vi "XYPlatform.vi"() -> ()   [LabVIEW 2017]
uses:
  <vilib>/Utility/error.llb/DialogType.ctl
  <vilib>/DAQmx/read.llb/DAQmx Read (Counter DBL 1Chan 1Samp).vi
  <vilib>/DAQmx/read.llb/DAQmx Read (Digital Bool 1Line 1Point).vi
  <vilib>/DAQmx/write.llb/DAQmx Write (Analog DBL 1Chan 1Samp).vi
  <vilib>/DAQmx/create/channels.llb/DAQmx Create Channel (AO-Voltage-Basic).vi
  <vilib>/DAQmx/create/channels.llb/DAQmx Create Channel (DI-Digital Input).vi
  <vilib>/DAQmx/create/channels.llb/DAQmx Create Channel (CI-Count Edges).vi
  <vilib>/functionblocks/Counter/Elapsed Timer/Elapsed Timer.vi
  <vilib>/DAQmx/miscellaneous.llb/DAQmx Fill In Error Info.vi
  <vilib>/functionblocks/FB Core/FB Core.xnode
  <vilib>/functionblocks/NI_FunctionBlock Libraries.lvlib
panel:
  in  "Zero":bool
  out "Dial Left Motor Voltage":dbl
  out "Dial Right Motor Voltage":dbl
  out "Left":bool
  out "Right":bool
  out "Down":bool
  out "Up":bool
  out "AngleLeft":bool
  out "RightIsStill":bool
  in  "Right Offset":dbl
  in  "Left Offset":dbl
  in  "Radius / cm":dbl
  out "Right Motor Pulses":dbl
  out "Left Motor Pulses":dbl
  in  "X position / cm":dbl(slide) scale=0.0..22.0
  in  "Y position / cm":dbl(slide) scale=0.0..14.0
  in  "Position Control":bool
  out "Y Position / cm":dbl
  out "X Position / cm":dbl
  in  "Draw Circle":bool
  out "Current Position":cluster{"Y":dbl[], "Y":dbl[]}[](graph)
  in  "X Voltage":dbl(slide) scale=-10.0..10.0
  in  "Y Voltage":dbl(slide) scale=-10.0..10.0
  in  "Home Button":bool=TRUE
  in  "Height / cm":dbl
  in  "Width / cm":dbl
  in  "Draw Rectangle":bool
  in  "Direction":sgl(knob)
  in  "Voltage of Dial":dbl
  out "Right Frequency (pulse/s)":dbl
  out "Left Frequency (pulse/s)":dbl
  out "Up Limit Switch":bool
  out "Down Limit Switch":bool
  out "Right Limit Switch":bool
  out "Left Limit Switch":bool
  in  "Left Motor Counter":tag="Dev5/ctr1"
  in  "Right Motor Counter":tag="Dev5/ctr0"
  in  "Left Limit Switch":tag="Dev5/port0/line3"
  in  "Right Limit Switch":tag="Dev5/port0/line2"
  in  "Down Limit Switch":tag="Dev5/port0/line1"
  in  "Up Limit Switch":tag="Dev5/port0/line0"
  in  "Motor Stop":bool
  in  "Left Motor":tag="Dev5/ao1"
  in  "Right Motor":tag="Dev5/ao0"
  in  "Min Voltage":dbl=-10.0
  in  "Max Voltage":dbl=10.0
  out "AngleRight":bool
  out "AngleDown":bool
  out "AngleUp":bool
  out "LeftIsStill":bool
  in  "Program Stop":bool
  out "Rectangle Right Ref":dbl
  out "Rectangle Left Ref":dbl
  out "Net Left Pulse":dbl
  out "Net Right Pulse":dbl
  out "Left Motor":dbl
  out "Right Motor":dbl
  out "Left Motor Pulses":dbl
  out "last left pulse":dbl format="%0.2f"
  out "Right Motor Pulses":dbl
  out "last right pulse":dbl format="%0.2f"
  out "Right Motor Timer":i32
  out "Left Motor Timer":i32
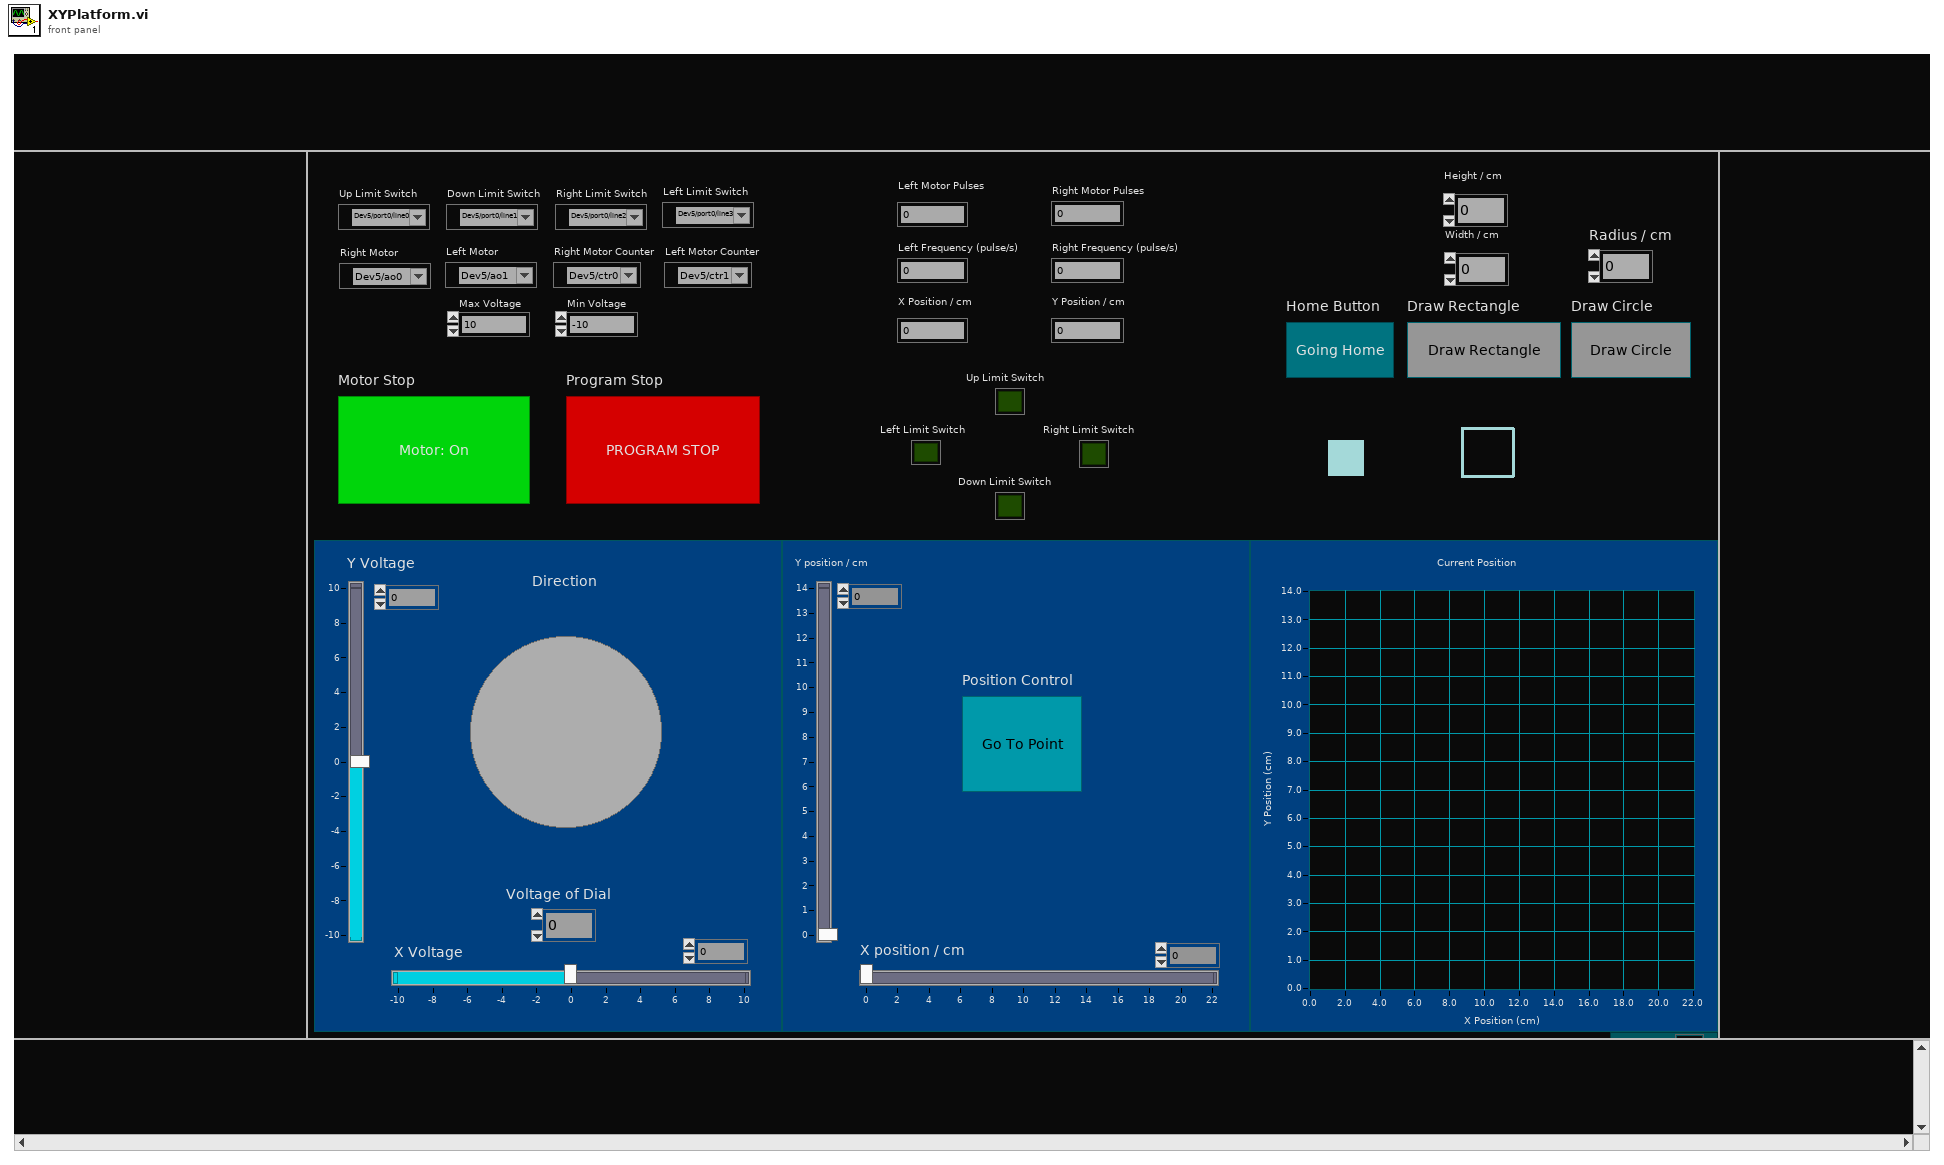
[diagram p1: front panel]
types:
  T1 = typedef "DialogType.ctl" = u16
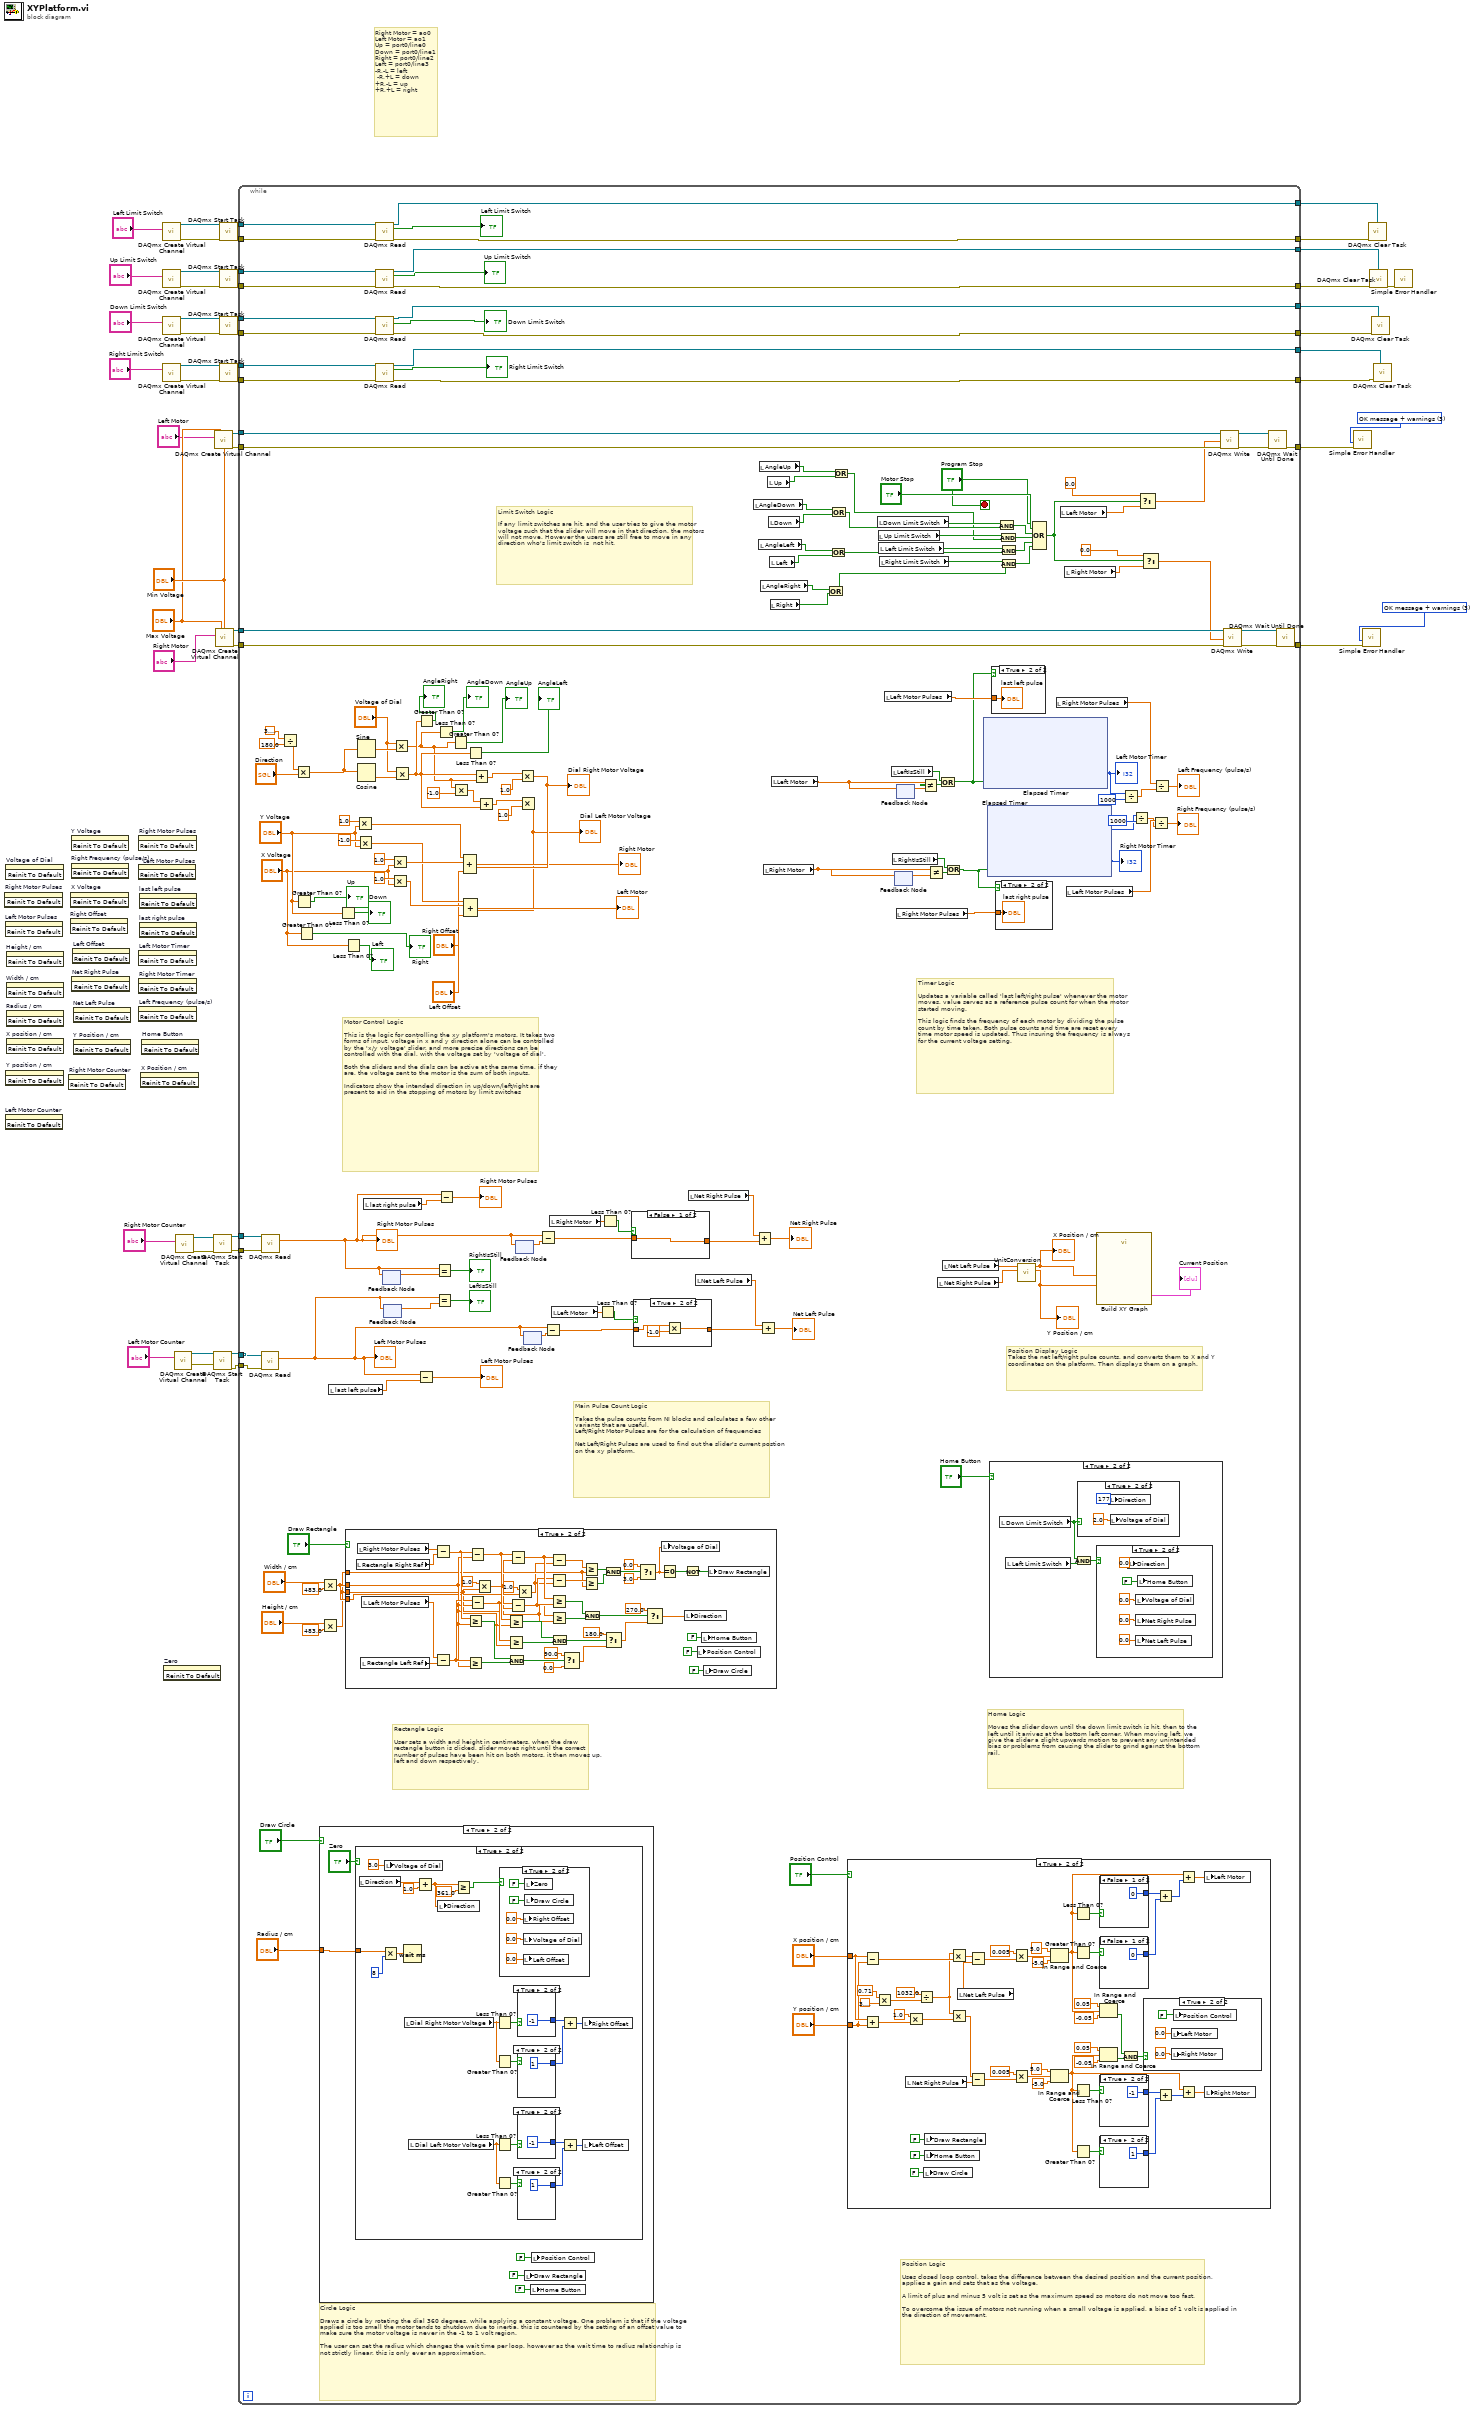
[diagram p0: block diagram]
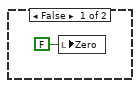
[diagram p2: hidden frame]
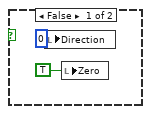
[diagram p3: hidden frame]
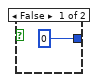
[diagram p5: hidden frame]
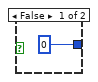
[diagram p6: hidden frame]
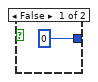
[diagram p7: hidden frame]
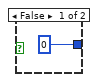
[diagram p8: hidden frame]
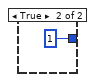
[diagram p11: hidden frame]
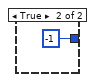
[diagram p12: hidden frame]
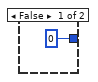
[diagram p13: hidden frame]
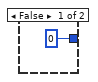
[diagram p14: hidden frame]
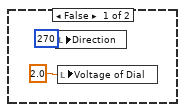
[diagram p17: hidden frame]
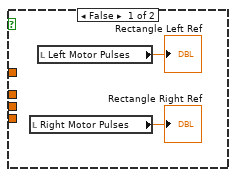
[diagram p18: hidden frame]
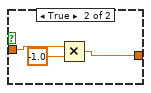
[diagram p20: hidden frame]
diagram:
  w11 = T1 3 items=["no dialog", "OK message", "continue or stop message", "OK message + warnings", "continue/stop + warnings"] ("type of dialog (OK msg:1)")
  w12 = T1 3 items=["no dialog", "OK message", "continue or stop message", "OK message + warnings", "continue/stop + warnings"] ("type of dialog (OK msg:1)")
  # "Right Motor = ao0\nLeft Motor = ao1\nUp = port0/line0 \nDown = port0/line1 \nRight = port0/line2\nLeft = port0/line3\n-R,-L = left\n -R,+L = down\n+R,-L = up\n+R,+L = right"
  n1 = invoke on="Right Motor Pulses" class="DigNum (strict)" method="Reinit To Default"() -> ()  [unwired: 3 in, 3 out]
  n2 = invoke on="Left Motor Pulses" class="DigNum (strict)" method="Reinit To Default"() -> ()  [unwired: 3 in, 3 out]
  n3 = invoke on="Left Motor Counter" class="DAQmxName" method="Reinit To Default"() -> ()  [unwired: 3 in, 3 out]
  n4 = invoke on="Voltage of Dial" class="DigNum (strict)" method="Reinit To Default"() -> ()  [unwired: 3 in, 3 out]
  n5 = invoke on="Y position / cm" class="Slide (strict)" method="Reinit To Default"() -> ()  [unwired: 3 in, 3 out]
  n6 = invoke on="Height / cm" class="DigNum (strict)" method="Reinit To Default"() -> ()  [unwired: 3 in, 3 out]
  n7 = invoke on="Width / cm" class="DigNum (strict)" method="Reinit To Default"() -> ()  [unwired: 3 in, 3 out]
  n8 = invoke on="Radius / cm" class="DigNum (strict)" method="Reinit To Default"() -> ()  [unwired: 3 in, 3 out]
  n9 = invoke on="X position / cm" class="Slide (strict)" method="Reinit To Default"() -> ()  [unwired: 3 in, 3 out]
  n10 = invoke on="Right Motor Counter" class="DAQmxName" method="Reinit To Default"() -> ()  [unwired: 3 in, 3 out]
  n11 = invoke on="Right Offset" class="DigNum (strict)" method="Reinit To Default"() -> ()  [unwired: 3 in, 3 out]
  n12 = invoke on="X Voltage" class="Slide (strict)" method="Reinit To Default"() -> ()  [unwired: 3 in, 3 out]
  n13 = invoke on="Y Voltage" class="Slide (strict)" method="Reinit To Default"() -> ()  [unwired: 3 in, 3 out]
  n14 = invoke on="Right Frequency (pulse/s)" class="DigNum (strict)" method="Reinit To Default"() -> ()  [unwired: 3 in, 3 out]
  n15 = invoke on="Net Right Pulse" class="DigNum (strict)" method="Reinit To Default"() -> ()  [unwired: 3 in, 3 out]
  n16 = invoke on="Left Offset" class="DigNum (strict)" method="Reinit To Default"() -> ()  [unwired: 3 in, 3 out]
  n17 = invoke on="Net Left Pulse" class="DigNum (strict)" method="Reinit To Default"() -> ()  [unwired: 3 in, 3 out]
  n18 = invoke on="Y Position / cm" class="DigNum (strict)" method="Reinit To Default"() -> ()  [unwired: 3 in, 3 out]
  n19 = invoke on="Left Motor Pulses" class="DigNum (strict)" method="Reinit To Default"() -> ()  [unwired: 3 in, 3 out]
  n20 = invoke on="Right Motor Pulses" class="DigNum (strict)" method="Reinit To Default"() -> ()  [unwired: 3 in, 3 out]
  n21 = invoke on="Left Motor Timer" class="DigNum (strict)" method="Reinit To Default"() -> ()  [unwired: 3 in, 3 out]
  n22 = invoke on="Right Motor Timer" class="DigNum (strict)" method="Reinit To Default"() -> ()  [unwired: 3 in, 3 out]
  n23 = invoke on="Left Frequency (pulse/s)" class="DigNum (strict)" method="Reinit To Default"() -> ()  [unwired: 3 in, 3 out]
  n24 = invoke on="last left pulse" class="DigNum (strict)" method="Reinit To Default"() -> ()  [unwired: 3 in, 3 out]
  n25 = invoke on="last right pulse" class="DigNum (strict)" method="Reinit To Default"() -> ()  [unwired: 3 in, 3 out]
  n26 = invoke on="X Position / cm" class="DigNum (strict)" method="Reinit To Default"() -> ()  [unwired: 3 in, 3 out]
  n27 = invoke on="Home Button" class="Bool (strict)" method="Reinit To Default"() -> ()  [unwired: 3 in, 3 out]
  n28 = call-poly <vilib>:"DAQmx Create Virtual Channel.vi"("lines"="Left Limit Switch") -> ("task out"=w35:refnum<k21>, "error out"=w34:errorcluster)  [unwired: 13 in]
  n29 = call-poly <vilib>:"DAQmx Create Virtual Channel.vi"("lines"="Up Limit Switch") -> ("task out"=w41:refnum<k21>, "error out"=w40:errorcluster)  [unwired: 13 in]
  n30 = call-poly <vilib>:"DAQmx Create Virtual Channel.vi"("lines"="Down Limit Switch") -> ("task out"=w39:refnum<k21>, "error out"=w38:errorcluster)  [unwired: 13 in]
  n31 = call-poly <vilib>:"DAQmx Create Virtual Channel.vi"("lines"="Right Limit Switch") -> ("task out"=w37:refnum<k21>, "error out"=w36:errorcluster)  [unwired: 13 in]
  n32 = invoke on="Zero" class="Bool (strict)" method="Reinit To Default"() -> ()  [unwired: 3 in, 3 out]
  n33 = call-poly <vilib>:"DAQmx Create Virtual Channel.vi"("counter"="Left Motor Counter") -> ("task out"=w8:refnum<k21>, "error out"=w5:errorcluster)  [unwired: 13 in]
  n34 = call-poly <vilib>:"DAQmx Create Virtual Channel.vi"("counter"="Right Motor Counter") -> ("task out"=w10:refnum<k21>, "error out"=w6:errorcluster)  [unwired: 13 in]
  n35 = call <vilib>:"DAQmx Start Task.vi"("task/channels in"=w10, "error in"=w6) -> ("task out"=w9:refnum<k21>, "error out"=w4:errorcluster)  [unwired: 12 in]
  n36 = call <vilib>:"DAQmx Start Task.vi"("task/channels in"=w8, "error in"=w5) -> ("task out"=w7:refnum<k21>, "error out"=w3:errorcluster)  [unwired: 12 in]
  n37 = call-poly <vilib>:"DAQmx Create Virtual Channel.vi"("maximum value"="Max Voltage", "minimum value"="Min Voltage", "physical channels"="Left Motor") -> ("task out"=w47:refnum<k21>, "error out"=w46:errorcluster)  [unwired: 11 in]
  n38 = call-poly <vilib>:"DAQmx Create Virtual Channel.vi"("maximum value"="Max Voltage", "minimum value"="Min Voltage", "physical channels"="Right Motor") -> ("task out"=w50:refnum<k21>, "error out"=w49:errorcluster)  [unwired: 11 in]
  n39 = call <vilib>:"DAQmx Start Task.vi"("task/channels in"=w35, "error in"=w34) -> ("task out"=w19:refnum<k21>, "error out"=w18:errorcluster)  [unwired: 12 in]
  n40 = call <vilib>:"DAQmx Start Task.vi"("task/channels in"=w41, "error in"=w40) -> ("task out"=w33:refnum<k21>, "error out"=w32:errorcluster)  [unwired: 12 in]
  n41 = call <vilib>:"DAQmx Start Task.vi"("task/channels in"=w39, "error in"=w38) -> ("task out"=w27:refnum<k21>, "error out"=w26:errorcluster)  [unwired: 12 in]
  n42 = call <vilib>:"DAQmx Start Task.vi"("task/channels in"=w37, "error in"=w36) -> ("task out"=w23:refnum<k21>, "error out"=w22:errorcluster)  [unwired: 12 in]
  n43 = while {
    tunnel: w50 -> [w218]
    tunnel: w49 -> [w216]
    tunnel: [w214] -> w48
    tunnel: w47 -> [w213]
    tunnel: w46 -> [w210]
    tunnel: [w209] -> w42
    tunnel: w33 -> [w206]
    tunnel: w32 -> [w205]
    tunnel: [w204] -> w31
    tunnel: [w203] -> w30
    tunnel: w27 -> [w202]
    tunnel: w26 -> [w201]
    tunnel: [w200] -> w25
    tunnel: w23 -> [w199]
    tunnel: w22 -> [w198]
    tunnel: [w197] -> w14
    tunnel: [w196] -> w21
    tunnel: w19 -> [w195]
    tunnel: w18 -> [w194]
    tunnel: [w193] -> w17
    tunnel: [w192] -> w16
    tunnel: w9 -> [w189]
    tunnel: w7 -> [w188]
    tunnel: [w187] -> w13
    tunnel: w4 -> [w176]
    tunnel: w3 -> [w175]
    stop <- "Program Stop" stop-if-true
    # "Position Logic\n\nUses closed loop control, takes the difference between the desired position and the current position, applies a gain and sets that as the voltage. \n\nA limit of plus and minus 5 volt is set as the maximum speed so motors do not move too fast. \n\nTo overcome the issue of motors not running when a small voltage is applied, a bias of 1 volt is applied in the direction of movement."
    # "Circle Logic\n\nDraws a circle by rotating the dial 360 degrees, while applying a constant voltage. One problem is that if the voltage applied is too small the motor tends to shutdown due to inertia, this is countered by the setting of an offset value to make sure the motor voltage is never in the -1 to 1 volt region.\n\nThe user can set the radius which changes the wait time per loop, however as the wait time to radius relationship is not strictly linear, this is only ever an approximation."
    # "Home Logic\n\nMoves the slider down until the down limit switch is hit, then to the left until it arrives at the bottom left corner. When moving left, we give the slider a slight upwards motion to prevent any unintended bias or problems from causing the slider to grind against the bottom rail."
    # "Rectangle Logic\n\nUser sets a width and height in centimeters, when the draw rectangle button is clicked, slider moves right until the correct number of pulses have been hit on both motors, it then moves up, left and down respectively."
    # "Position Display Logic\nTakes the net left/right pulse counts, and converts them to X and Y coordinates on the platform. Then displays them on a graph."
    # "Main Pulse Count Logic\n\nTakes the pulse counts from NI blocks and calculates a few other variants that are useful. \nLeft/Right Motor Pulses are for the calculation of frequencies\n\nNet Left/Right Pulses are used to find out the slider's current postion on the xy platform."
    # "Limit Switch Logic\n\nIf any limit switches are hit, and the user tries to give the motor voltage such that the slider will move in that direction, the motors will not move. However the users are still free to move in any direction who's limit switch is  not hit."
    # "Motor Control Logic\n\nThis is the logic for controlling the xy platform's motors. It takes two forms of input, voltage in x and y direction alone can be controlled by the 'x/y voltage' slider, and more precise directions can be controlled with the dial, with the voltage set by 'voltage of dial'.\n\nBoth the sliders and the dials can be active at the same time, if they are, the voltage sent to the motor is the sum of both inputs.\n\nIndicators show the intended direction in up/down/left/right are present to aid in the stopping of motors by limit switches"
    # "Timer Logic\n\nUpdates a variable called 'last left/right pulse' whenever the motor moves, value serves as a reference pulse count for when the motor started moving.\n\nThis logic finds the frequency of each motor by dividing the pulse count by time taken. Both pulse counts and time are reset every time motor speed is updated. Thus insuring the frequency is always for the current voltage setting."
    n44 = call-poly <vilib>:"DAQmx Read.vi"("task/channels in"=w188, "error in"=w175) -> ("data"=w73:dbl)  [unwired: 11 in, 2 out]
    "Left Motor Pulses" <- w73
    n45 = call-poly <vilib>:"DAQmx Read.vi"("task/channels in"=w189, "error in"=w176) -> ("data"=w115:dbl)  [unwired: 11 in, 2 out]
    "Right Motor Pulses" <- w115
    n46 = Divide(x=3.141592653589793, y=180.0) -> (x/y=w109:dbl)
    n47 = Multiply(x=w109, y="Direction") -> (x*y=w112:dbl)
    n48 = Greater Than 0?(x="Y Voltage") -> (x > 0?=→"Up":bool)
    n49 = Greater Than 0?(x="X Voltage") -> (x > 0?=→"Right":bool)
    n50 = case shown="True" "Draw Circle" {
      tunnel: "Radius / cm" -> [_ w223]
      frame False {
        n51 = local write "Zero"(FALSE ("Zero")) -> ()
      }
      frame True {
        n52 = case shown="True" "Zero" {
          tunnel: w223 -> [_ w227]
          frame False {
            n53 = local write "Direction"(u16 0 ("Dial")) -> ()
            n54 = local write "Zero"(TRUE ("Zero")) -> ()
          }
          frame True {
            n55 = local read "Direction"() -> (w246:sgl)
            n56 = Multiply(x=w227, y=u32 8 ("milliseconds to wait")) -> (x*y=w229:dbl)
            n57 = local write "Voltage of Dial"(3.0 ("Voltage of Dial")) -> ()
            n58 = Wait (ms)(milliseconds to wait=w229) -> ()  [unwired: 1 out]
            n59 = local read "Dial Right Motor Voltage"() -> (w232:dbl)
            n60 = local read "Dial Left Motor Voltage"() -> (w231:dbl)
            n61 = Add(x=w246, y=1.0) -> (x+y=w245:dbl)
            n62 = local write "Direction"(w245) -> ()
            n63 = Greater Or Equal?(x=w245, y=361.0) -> (x >= y?=w230:bool)
            n64 = Less Than 0?(x=w232) -> (x < 0?=w240:bool)
            n65 = Greater Than 0?(x=w232) -> (x > 0?=w239:bool)
            n66 = Less Than 0?(x=w231) -> (x < 0?=w242:bool)
            n67 = Greater Than 0?(x=w231) -> (x > 0?=w241:bool)
            n68 = case shown="True" w230 {
              frame False {
              }
              frame True {
                n69 = local write "Right Offset"(0.0 ("Right Offset")) -> ()
                n70 = local write "Voltage of Dial"(0.0 ("Voltage of Dial")) -> ()
                n71 = local write "Left Offset"(0.0 ("Left Offset")) -> ()
                n72 = local write "Zero"(FALSE ("Zero")) -> ()
                n73 = local write "Draw Circle"(FALSE ("Draw Circle")) -> ()
              }
            }
            n74 = case shown="True" w240 {
              tunnel: [0 -1] -> w235
              frame False {
              }
              frame True {
              }
            }
            n75 = case shown="True" w239 {
              tunnel: [0 1] -> w234
              frame False {
              }
              frame True {
              }
            }
            n76 = case shown="True" w242 {
              tunnel: [0 -1] -> w238
              frame False {
              }
              frame True {
              }
            }
            n77 = case shown="True" w241 {
              tunnel: [0 1] -> w237
              frame False {
              }
              frame True {
              }
            }
            n78 = Add(x=w235, y=w234) -> (x+y=w233:i32)
            n79 = Add(x=w238, y=w237) -> (x+y=w236:i32)
            n80 = local write "Right Offset"(w233) -> ()
            n81 = local write "Left Offset"(w236) -> ()
          }
        }
        n82 = local write "Draw Rectangle"(FALSE ("Draw Rectangle")) -> ()
        n83 = local write "Home Button"(FALSE ("Home Button")) -> ()
        n84 = local write "Position Control"(FALSE ("Position Control")) -> ()
      }
    }
    n85 = Multiply(x="Width / cm", y=483.0) -> (x*y=w57:dbl)
    n86 = Multiply(x="Height / cm", y=483.0) -> (x*y=w54:dbl)
    n87 = local read "last left pulse"() -> (w170:dbl)
    n88 = Less Than 0?(x="Y Voltage") -> (x < 0?=→"Down":bool)
    n89 = Less Than 0?(x="X Voltage") -> (x < 0?=→"Left":bool)
    n90 = case shown="True" "Draw Rectangle" {
      tunnel: w57 -> [_ w361]
      tunnel: w54 -> [_ w339]
      tunnel: w57 -> [_ w343]
      tunnel: w54 -> [_ w352]
      frame False {
        n91 = local read "Right Motor Pulses"() -> (→"Rectangle Right Ref":dbl)
        n92 = local read "Left Motor Pulses"() -> (→"Rectangle Left Ref":dbl)
      }
      frame True {
        n93 = local read "Rectangle Right Ref"() -> (w378:dbl)
        n94 = local read "Right Motor Pulses"() -> (w379:dbl)
        n95 = local read "Rectangle Left Ref"() -> (w376:dbl)
        n96 = local read "Left Motor Pulses"() -> (w377:dbl)
        n97 = Subtract(x=w379, y=w378) -> (x-y=w370:dbl)
        n98 = Subtract(x=w377, y=w376) -> (x-y=w369:dbl)
        n99 = Greater Or Equal?(x=w370, y=w361) -> (x >= y?=w374:bool)
        n100 = Greater Or Equal?(x=w369, y=w361) -> (x >= y?=w375:bool)
        n101 = Subtract(x=w370, y=w361) -> (x-y=w363:dbl)
        n102 = Subtract(x=w369, y=w361) -> (x-y=w362:dbl)
        n103 = Multiply(x=1.0, y=w339) -> (x*y=w338:dbl)
        n104 = Greater Or Equal?(x=w363, y=w339) -> (x >= y?=w368:bool)
        n105 = Greater Or Equal?(x=w362, y=w339) -> (x >= y?=w367:bool)
        n106 = And(x=w374, y=w375) -> (x .and. y?=w373:bool)
        n107 = Subtract(x=w363, y=w338) -> (x-y=w356:dbl)
        n108 = Subtract(x=w362, y=w338) -> (x-y=w355:dbl)
        n109 = Multiply(x=1.0, y=w343) -> (x*y=w341:dbl)
        n110 = Subtract(x=w356, y=w341) -> (x-y=w354:dbl)
        n111 = Subtract(x=w355, y=w341) -> (x-y=w353:dbl)
        n112 = Greater Or Equal?(x=w356, y=w361) -> (x >= y?=w360:bool)
        n113 = Greater Or Equal?(x=w355, y=w361) -> (x >= y?=w359:bool)
        n114 = And(x=w368, y=w367) -> (x .and. y?=w366:bool)
        n115 = Select(t=90.0, s=w373, f=0.0) -> (s? t:f=w371:dbl)
        n116 = Greater Or Equal?(x=w354, y=w352) -> (x >= y?=w351:bool)
        n117 = Greater Or Equal?(x=w353, y=w352) -> (x >= y?=w350:bool)
        n118 = And(x=w360, y=w359) -> (x .and. y?=w358:bool)
        n119 = And(x=w351, y=w350) -> (x .and. y?=w349:bool)
        n120 = Select(t=180.0, s=w366, f=w371) -> (s? t:f=w364:dbl)
        n121 = Select(t=0.0, s=w349, f=3.0) -> (s? t:f=w346:dbl)
        n122 = Select(t=270.0, s=w358, f=w364) -> (s? t:f=w357:dbl)
        n123 = Equal To 0?(x=w346) -> (x = 0?=w345:bool)
        n124 = local write "Voltage of Dial"(w346) -> ()
        n125 = Not(x=w345) -> (.not. x?=w344:bool)
        n126 = local write "Direction"(w357) -> ()
        n127 = local write "Position Control"(FALSE ("Position Control")) -> ()
        n128 = local write "Home Button"(FALSE ("Home Button")) -> ()
        n129 = local write "Draw Circle"(FALSE ("Draw Circle")) -> ()
        n130 = local write "Draw Rectangle"(w344) -> ()
      }
    }
    n131 = Multiply(x=1.0, y="Y Voltage") -> (x*y=w102:dbl)
    n132 = Multiply(x=-1.0, y="Y Voltage") -> (x*y=w103:dbl)
    n133 = Cosine(x=w112) -> (cos(x)=w129:dbl)
    n134 = Sine(x=w112) -> (sin(x)=w128:dbl)
    n135 = local read "last right pulse"() -> (w173:dbl)
    n136 = call-poly <vilib>:"DAQmx Read.vi"("task/channels in"=w195, "error in"=w194) -> ("task out"=w193:refnum<k21>, "data"=→"Left Limit Switch":bool, "error out"=w192:errorcluster)  [unwired: 11 in]
    n137 = call-poly <vilib>:"DAQmx Read.vi"("task/channels in"=w206, "error in"=w205) -> ("task out"=w204:refnum<k21>, "data"=→"Up Limit Switch":bool, "error out"=w203:errorcluster)  [unwired: 11 in]
    n138 = call-poly <vilib>:"DAQmx Read.vi"("task/channels in"=w202, "error in"=w201) -> ("task out"=w187:refnum<k21>, "data"=→"Down Limit Switch":bool, "error out"=w200:errorcluster)  [unwired: 11 in]
    n139 = call-poly <vilib>:"DAQmx Read.vi"("task/channels in"=w199, "error in"=w198) -> ("task out"=w197:refnum<k21>, "data"=→"Right Limit Switch":bool, "error out"=w196:errorcluster)  [unwired: 11 in]
    n140 = feedback #1() -> (w163:dbl)  [unwired: 1 in]
    n141 = feedback-in #1(w115) -> ()
    n142 = feedback #2() -> (w162:dbl)  [unwired: 1 in]
    n143 = feedback-in #2(w73) -> ()
    n144 = Multiply(x=1.0, y="X Voltage") -> (x*y=w127:dbl)
    n145 = Multiply(x=1.0, y="X Voltage") -> (x*y=w126:dbl)
    n146 = Multiply(x="Voltage of Dial", y=w128) -> (x*y=w131:dbl)
    n147 = Multiply(x="Voltage of Dial", y=w129) -> (x*y=w132:dbl)
    n148 = Subtract(x=w73, y=w170) -> (x-y=→"Left Motor Pulses":dbl)
    n149 = Greater Than 0?(x=w132) -> (x > 0?=→"AngleRight":bool)
    n150 = Equal?(x=w115, y=w163) -> (x = y?=→"RightIsStill":bool)
    n151 = Equal?(x=w73, y=w162) -> (x = y?=→"LeftIsStill":bool)
    n152 = Less Than 0?(x=w131) -> (x < 0?=→"AngleDown":bool)
    n153 = Subtract(x=w115, y=w173) -> (x-y=→"Right Motor Pulses":dbl)
    n154 = Greater Than 0?(x=w131) -> (x > 0?=→"AngleUp":bool)
    n155 = Multiply(x=w131, y=-1.0) -> (x*y=w130:dbl)
    n156 = Less Than 0?(x=w132) -> (x < 0?=→"AngleLeft":bool)
    n157 = Add(x=w132, y=w131) -> (x+y=w108:dbl)
    n158 = Add(x=w130, y=w132) -> (x+y=w107:dbl)
    n159 = feedback-in #3(w115) -> ()
    n160 = feedback #3() -> (w143:dbl)  [unwired: 1 in]
    n161 = Multiply(x=w108, y=1.0) -> (x*y=w104:dbl)
    "Dial Right Motor Voltage" <- w104
    n162 = Compound Arithmetic op=ADD(w102, w127, w104, "Right Offset") -> (→"Right Motor":dbl)
    n163 = Multiply(x=w107, y=1.0) -> (x*y=w97:dbl)
    "Dial Left Motor Voltage" <- w97
    n164 = Compound Arithmetic op=ADD(w103, w126, w97, "Left Offset") -> (→"Left Motor":dbl)
    n165 = feedback #4() -> (w142:dbl)  [unwired: 1 in]
    n166 = feedback-in #4(w73) -> ()
    n167 = Subtract(x=w115, y=w143) -> (x-y=w72:dbl)
    n168 = Subtract(x=w73, y=w142) -> (x-y=w71:dbl)
    n169 = local read "Right Motor"() -> (w141:dbl)
    n170 = local read "Left Motor"() -> (w139:dbl)
    n171 = Less Than 0?(x=w139) -> (x < 0?=w138:bool)
    n172 = Less Than 0?(x=w141) -> (x < 0?=w140:bool)
    n173 = case shown="False" w140 {
      tunnel: w72 -> [w386 w389]
      tunnel: [w386 w388] -> w69
      frame False {
      }
      frame True {
        n174 = Multiply(x=w389, y=-1.0) -> (x*y=w388:dbl)
      }
    }
    n175 = case shown="True" w138 {
      tunnel: w71 -> [w382 w384]
      tunnel: [w382 w385] -> w70
      frame False {
      }
      frame True {
        n176 = Multiply(x=w384, y=-1.0) -> (x*y=w385:dbl)
      }
    }
    n177 = local read "Net Right Pulse"() -> (w136:dbl)
    n178 = local read "Net Left Pulse"() -> (w134:dbl)
    n179 = local read "AngleDown"() -> (w84:bool)
    n180 = Add(x=w136, y=w69) -> (x+y=→"Net Right Pulse":dbl)
    n181 = local read "AngleLeft"() -> (w120:bool)
    n182 = local read "AngleUp"() -> (w121:bool)
    n183 = Add(x=w134, y=w70) -> (x+y=→"Net Left Pulse":dbl)
    n184 = local read "AngleRight"() -> (w85:bool)
    n185 = local read "Right Motor"() -> (w147:dbl)
    n186 = local read "Up"() -> (w81:bool)
    n187 = local read "Down"() -> (w83:bool)
    n188 = local read "Left"() -> (w82:bool)
    n189 = local read "Right"() -> (w86:bool)
    n190 = local read "Left Motor"() -> (w146:dbl)
    n191 = Or(x=w85, y=w86) -> (x .or. y?=w116:bool)
    n192 = Or(x=w120, y=w82) -> (x .or. y?=w117:bool)
    n193 = Or(x=w84, y=w83) -> (x .or. y?=w119:bool)
    n194 = Or(x=w121, y=w81) -> (x .or. y?=w118:bool)
    n195 = case shown="True" "Position Control" {
      tunnel: "X position / cm" -> [_ w303]
      tunnel: "Y position / cm" -> [_ w302]
      frame False {
      }
      frame True {
        n196 = Subtract(x=w303, y=w302) -> (x-y=w300:dbl)
        n197 = Add(x=w303, y=w302) -> (x+y=w305:dbl)
        n198 = Multiply(x=0.71, y=3.141592653589793) -> (x*y=w308:dbl)
        n199 = local read "Net Right Pulse"() -> (w295:dbl)
        n200 = Multiply(x=1.0, y=w305) -> (x*y=w301:dbl)
        n201 = Divide(x=1032.0, y=w308) -> (x/y=w299:dbl)
        n202 = local write "Draw Circle"(FALSE ("Draw Circle")) -> ()
        n203 = local write "Draw Rectangle"(FALSE ("Draw Rectangle")) -> ()
        n204 = local write "Home Button"(FALSE ("Home Button")) -> ()
        n205 = Multiply(x=w299, y=w300) -> (x*y=w298:dbl)
        n206 = Multiply(x=w299, y=w301) -> (x*y=w296:dbl)
        n207 = local read "Net Left Pulse"() -> (w297:dbl)
        n208 = Subtract(x=w298, y=w297) -> (x-y=w294:dbl)
        n209 = Subtract(x=w296, y=w295) -> (x-y=w293:dbl)
        n210 = Multiply(x=0.005, y=w294) -> (x*y=w290:dbl)
        n211 = Multiply(x=0.005, y=w293) -> (x*y=w287:dbl)
        n212 = In Range and Coerce(upper limit=5.0, x=w290, lower limit=-5.0) -> (coerced(x)=w266:dbl)  [unwired: 1 out]
        n213 = In Range and Coerce(upper limit=5.0, x=w287, lower limit=-5.0) -> (coerced(x)=w265:dbl)  [unwired: 1 out]
        n214 = Less Than 0?(x=w266) -> (x < 0?=w282:bool)
        n215 = Greater Than 0?(x=w266) -> (x > 0?=w281:bool)
        n216 = Less Than 0?(x=w265) -> (x < 0?=w284:bool)
        n217 = Greater Than 0?(x=w265) -> (x > 0?=w283:bool)
        n218 = case shown="False" w282 {
          tunnel: [0 -1] -> w280
          frame False {
          }
          frame True {
          }
        }
        n219 = case shown="False" w281 {
          tunnel: [0 1] -> w279
          frame False {
          }
          frame True {
          }
        }
        n220 = case shown="True" w284 {
          tunnel: [0 -1] -> w278
          frame False {
          }
          frame True {
          }
        }
        n221 = case shown="True" w283 {
          tunnel: [0 1] -> w277
          frame False {
          }
          frame True {
          }
        }
        n222 = In Range and Coerce(upper limit=0.05, x=w266, lower limit=-0.05) -> (In Range?=w268:bool)  [unwired: 1 out]
        n223 = In Range and Coerce(upper limit=0.05, x=w265, lower limit=-0.05) -> (In Range?=w267:bool)  [unwired: 1 out]
        n224 = And(x=w268, y=w267) -> (x .and. y?=w264:bool)
        n225 = case shown="True" w264 {
          frame False {
          }
          frame True {
            n226 = local write "Left Motor"(0.0 ("Left Motor")) -> ()
            n227 = local write "Right Motor"(0.0 ("Right Motor")) -> ()
            n228 = local write "Position Control"(FALSE ("Go 2")) -> ()
          }
        }
        n229 = Add(x=w280, y=w279) -> (x+y=w276:i32)
        n230 = Add(x=w278, y=w277) -> (x+y=w275:i32)
        n231 = Add(x=w266, y=w276) -> (x+y=w273:dbl)
        n232 = Add(x=w265, y=w275) -> (x+y=w274:dbl)
        n233 = local write "Left Motor"(w273) -> ()
        n234 = local write "Right Motor"(w274) -> ()
      }
    }
    n235 = local read "Down Limit Switch"() -> (w151:bool)
    n236 = local read "Up Limit Switch"() -> (w150:bool)
    n237 = local read "Left Limit Switch"() -> (w153:bool)
    n238 = local read "Right Limit Switch"() -> (w152:bool)
    n239 = local read "Left Motor Pulses"() -> (w171:dbl)
    n240 = local read "LeftIsStill"() -> (w149:bool)
    n241 = local read "RightIsStill"() -> (w148:bool)
    n242 = feedback #5() -> (w174:dbl)  [unwired: 1 in]
    n243 = feedback-in #5(w147) -> ()
    n244 = feedback-in #6(w146) -> ()
    n245 = feedback #6() -> (w177:dbl)  [unwired: 1 in]
    n246 = local read "Right Motor Pulses"() -> (w172:dbl)
    n247 = Not Equal?(x=w146, y=w177) -> (x != y?=w157:bool)
    n248 = Not Equal?(x=w147, y=w174) -> (x != y?=w156:bool)
    n249 = local read "Net Right Pulse"() -> (w65:dbl)
    n250 = Or(x=w149, y=w157) -> (x .or. y?=w159:bool)
    n251 = local read "Net Left Pulse"() -> (w66:dbl)
    n252 = Or(x=w148, y=w156) -> (x .or. y?=w158:bool)
    n253 = xnode "Elapsed Timer"("reset"=w159) -> ("elapsed time (ms)"=w79:i32)  [unwired: 2 in, 1 out]
    "Left Motor Timer" <- w79
    n254 = xnode "Elapsed Timer"("reset"=w158) -> ("elapsed time (ms)"=w75:i32)  [unwired: 2 in, 1 out]
    "Right Motor Timer" <- w75
    n255 = case shown="True" "Home Button" {
      frame False {
      }
      frame True {
        n256 = local read "Down Limit Switch"() -> (w322:bool)
        n257 = local read "Left Limit Switch"() -> (w321:bool)
        n258 = And(x=w322, y=w321) -> (x .and. y?=w323:bool)
        n259 = case shown="True" w322 {
          frame False {
            n260 = local write "Direction"(u16 270 ("Dial")) -> ()
            n261 = local write "Voltage of Dial"(2.0 ("Voltage of Dial")) -> ()
          }
          frame True {
            n262 = local write "Direction"(u16 177 ("Dial")) -> ()
            n263 = local write "Voltage of Dial"(2.0 ("Voltage of Dial")) -> ()
          }
        }
        n264 = case shown="True" w323 {
          frame False {
          }
          frame True {
            n265 = local write "Direction"(0.0 ("Net Right Pulse")) -> ()
            n266 = local write "Voltage of Dial"(0.0 ("Net Left Pulse")) -> ()
            n267 = local write "Net Right Pulse"(0.0 ("Y")) -> ()
            n268 = local write "Net Left Pulse"(0.0 ("X")) -> ()
            n269 = local write "Home Button"(FALSE ("Home Button")) -> ()
          }
        }
      }
    }
    n270 = case shown="True" w159 {
      tunnel: w171 -> [_ w390]
      frame False {
      }
      frame True {
        "last left pulse" <- w390
      }
    }
    n271 = case shown="True" w158 {
      tunnel: w172 -> [_ w391]
      frame False {
      }
      frame True {
        "last right pulse" <- w391
      }
    }
    n272 = And(x=w151, y=w119) -> (x .and. y?=w186:bool)
    n273 = And(x=w150, y=w118) -> (x .and. y?=w185:bool)
    n274 = And(x=w153, y=w117) -> (x .and. y?=w184:bool)
    n275 = And(x=w152, y=w116) -> (x .and. y?=w183:bool)
    n276 = call "UnitConversion.vi"("Net Right Pulse"=w65, "Net Left Pulse"=w66) -> ("X"=w53:dbl, "Y"=w52:dbl)  [unwired: 8 in]
    "X Position / cm" <- w52
    "Y Position / cm" <- w53
    n277 = Compound Arithmetic op=OR("Program Stop", "Motor Stop", w186, w185, w184, w183) -> (w181:bool)
    n278 = local read "Right Motor Pulses"() -> (w165:dbl)
    n279 = local read "Left Motor"() -> (w144:dbl)
    n280 = local read "Right Motor"() -> (w145:dbl)
    n281 = local read "Left Motor Pulses"() -> (w164:dbl)
    n282 = call "Build XY Graph"("Y Input"=w53, "X Input"=w52) -> ("XY Graph"=→"Current Position":cluster{"X":dbl[], "Y":dbl[]}[])  [unwired: 8 in, 1 out]
    n283 = Divide(x=w79, y=1000) -> (x/y=w78:dbl)
    n284 = Divide(x=w75, y=1000) -> (x/y=w74:dbl)
    n285 = Select(t=0.0 ("f"), s=w181, f=w144) -> (s? t:f=w207:dbl)
    n286 = Select(t=0.0 ("f"), s=w181, f=w145) -> (s? t:f=w208:dbl)
    n287 = Divide(x=w164, y=w74) -> (x/y=→"Right Frequency (pulse/s)":dbl)
    n288 = Divide(x=w165, y=w78) -> (x/y=→"Left Frequency (pulse/s)":dbl)
    n289 = call-poly <vilib>:"DAQmx Write.vi"("task/channels in"=w213, "data"=w207, "error in"=w210) -> ("task out"=w212:refnum<k21>, "error out"=w211:errorcluster)  [unwired: 10 in, 1 out]
    n290 = call-poly <vilib>:"DAQmx Write.vi"("task/channels in"=w218, "data"=w208, "error in"=w216) -> ("task out"=w217:refnum<k21>, "error out"=w215:errorcluster)  [unwired: 10 in, 1 out]
    n291 = call <vilib>:"DAQmx Wait Until Done.vi"("task/channels in"=w212, "error in"=w211) -> ("error out"=w209:errorcluster)  [unwired: 12 in, 1 out]
    n292 = call <vilib>:"DAQmx Wait Until Done.vi"("task/channels in"=w217, "error in"=w215) -> ("error out"=w214:errorcluster)  [unwired: 12 in, 1 out]
  }
  n293 = call <vilib>:"Simple Error Handler.vi"("type of dialog (OK msg:1)"=w11, "error in (no error)"=w42) -> ()  [unwired: 3 in, 5 out]
  n294 = call <vilib>:"Simple Error Handler.vi"("type of dialog (OK msg:1)"=w12, "error in (no error)"=w48) -> ()  [unwired: 3 in, 5 out]
  n295 = call <vilib>:"DAQmx Clear Task.vi"("task in"=w17, "error in"=w16) -> ()  [unwired: 13 in, 1 out]
  n296 = call <vilib>:"DAQmx Clear Task.vi"("task in"=w31, "error in"=w30) -> ("error out"=w15:errorcluster)  [unwired: 13 in]
  n297 = call <vilib>:"DAQmx Clear Task.vi"("task in"=w13, "error in"=w25) -> ()  [unwired: 13 in, 1 out]
  n298 = call <vilib>:"DAQmx Clear Task.vi"("task in"=w14, "error in"=w21) -> ()  [unwired: 13 in, 1 out]
  n299 = call <vilib>:"Simple Error Handler.vi"("error in (no error)"=w15) -> ()  [unwired: 4 in, 5 out]
